vi "Test 3.vi"   [LabVIEW 2021, in "Memory Map.lvclass"]
uses:
  Memory Map.lvclass
  <vilib>/addons/_JKI Toolkits/Caraya/classes/Assert/Assert True.vi
  <vilib>/addons/_JKI Toolkits/Caraya/classes/Assert/Assert False.vi
  <vilib>/addons/_JKI Toolkits/Caraya/classes/Test/Test.lvclass
  <vilib>/addons/_JKI Toolkits/Caraya/classes/Assert/Assert.lvclass
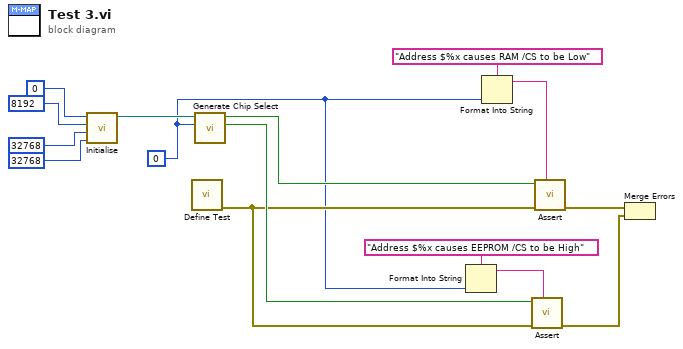
[diagram p0: block diagram]
diagram:
  w1 = u16 0 ("RAM Base Address")
  n1 = call "Initialise.vi"("EEPROM Size"=u16 32768 ("RAM Base Address"), "EEPROM Base Address"=u16 32768 ("RAM Base Address"), "RAM Size"=u16 8192 ("RAM Base Address"), "RAM Base Address"=u16 0) -> ("Memory Map out"=w11:refnum<class "Memory Map.lvclass">)  [unwired: 7 in]
  n2 = call <vilib>:"Define Test.vi"() -> ("error out"=w8:errorcluster)  [unwired: 11 in]
  n3 = call "Generate Chip Select.vi"("Address"=w1, "Memory Map in"=w11) -> ("EEPROM /CS"=w9:bool, "RAM /CS"=w10:bool)  [unwired: 8 in]
  n4 = Format Into String(format string="Address $%x causes EEPROM /CS to be High" ("Label"), w1) -> (resulting string=w2:string)  [unwired: 2 in, 1 out]
  n5 = Format Into String(format string="Address $%x causes RAM /CS to be Low" ("Label"), w1) -> (resulting string=w4:string)  [unwired: 2 in, 1 out]
  n6 = call-poly <vilib>:"Assert.vi"("Label"=w2, "error in (no error)"=w8, "True?"=w9) -> ("error out"=w6:errorcluster)  [unwired: 8 in]
  n7 = call-poly <vilib>:"Assert.vi"("Label"=w4, "error in (no error)"=w8, "False?"=w10) -> ("error out"=w7:errorcluster)  [unwired: 8 in]
  n8 = Merge Errors(w7, w6) -> ()  [unwired: 1 out]
